vi "disable.vi"(8 "error in (no error)":errorcluster, 11 "Stimulator090724Scaffold in":refnum<class "Stimulator090724Scaffold.lvclass">) -> (0 "error out":errorcluster, 3 "Stimulator090724Scaffold out":refnum<class "Stimulator090724Scaffold.lvclass">)   [LabVIEW 2010, in "Stimulator090724Scaffold.lvclass"]
uses:
  Stimulator090724Scaffold.lvclass
  Stimulator090724Scaffold.lvclass/Stimulator090724Scaffold.ctl
  Clock/GenericClock/GenericClock/GenericClock.lvclass
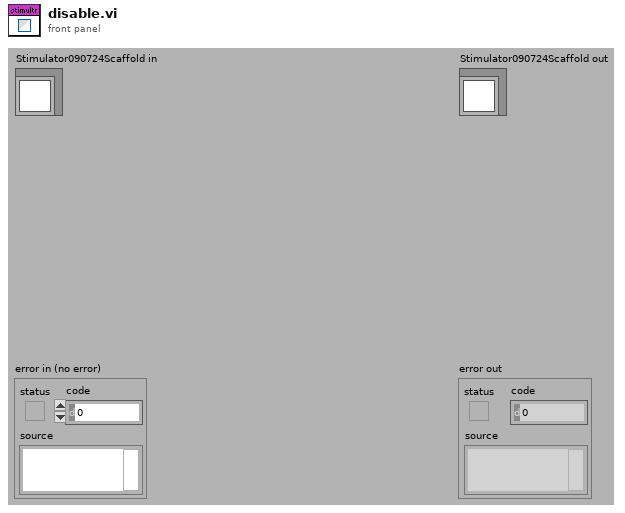
[diagram p1: front panel]
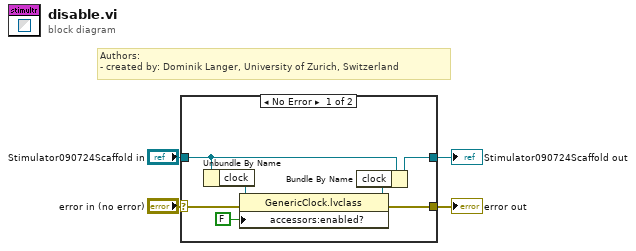
[diagram p0: block diagram]
diagram:
  # "Authors: \n- created by: Dominik Langer, University of Zurich, Switzerland"
  n1 = case shown="No Error" "error in (no error)" {
    selector: "error in (no error)" -> [w9 w12]
    tunnel: "Stimulator090724Scaffold in" -> [w7 w13]
    tunnel: [w8 w12] -> w2
    tunnel: [w6 w13] -> w1
    frame No Error {
      n2 = Unbundle By Name(w7) -> ("clock"=w11:refnum<class "GenericClock.lvclass">)
      n3 = property class="GenericClock.lvclass"(reference=w11, error in=w9, "accessors:enabled?"=FALSE ("enabled?")) -> (reference out=w10:refnum<class "GenericClock.lvclass">, error out=w8:errorcluster)
      n4 = Bundle By Name(cluster=w7, "clock"=w10) -> (w6:refnum<class "Stimulator090724Scaffold.lvclass">)
    }
    frame Error {
    }
  }
  "error out" <- w2
  "Stimulator090724Scaffold out" <- w1
